vi "Client.vi"() -> ()   [LabVIEW 2020]
panel:
  out "Data transmise":string
  out "bytes written 2":i32
  in  "Port distant":u16
  out "bytes written":i32
  in  "Vit":dbl(slide) scale=-1.0..1.0
  in  "stop":bool
  out "error out":errorcluster
  # "Client"
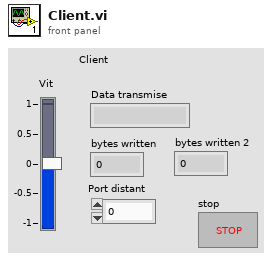
[diagram p1: front panel]
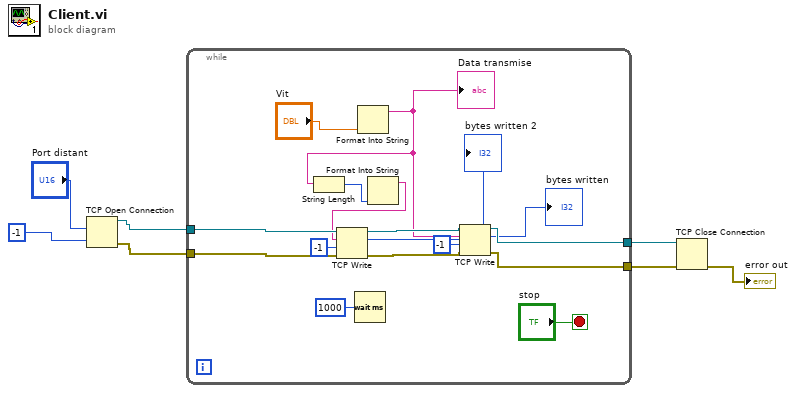
[diagram p0: block diagram]
diagram:
  n1 = TCP Open Connection(remote port or service name="Port distant", timeout ms (60000)=-1 ("timeout ms (wait forever: -1)")) -> (connection ID=w3:refnum<k5>, error out=w2:errorcluster)  [unwired: 3 in]
  n2 = while {
    tunnel: w3 -> [w21]
    tunnel: [w17] -> w7
    tunnel: w2 -> [w20]
    tunnel: [w18] -> w6
    stop <- "stop" stop-if-true
    n3 = Wait (ms)(milliseconds to wait=u32 1000) -> ()  [unwired: 1 out]
    n4 = Format Into String("Vit") -> (resulting string=w15:string)  [unwired: 3 in, 1 out]
    "Data transmise" <- w15
    n5 = String Length(string=w15) -> (length=w14:i32)
    n6 = Format Into String(w14) -> (resulting string=w8:string)  [unwired: 3 in, 1 out]
    n7 = TCP Write(connection ID=w21, data in=w8, error in (no error)=w20, 9:-1 ("timeout ms (25000)")) -> (connection ID out=w16:refnum<k5>, bytes written=→"bytes written 2":i32, error out=w19:errorcluster)
    n8 = TCP Write(connection ID=w16, data in=w15, error in (no error)=w19, 9:-1 ("timeout ms (25000)")) -> (connection ID out=w17:refnum<k5>, bytes written=→"bytes written":i32, error out=w18:errorcluster)
  }
  n9 = TCP Close Connection(connection ID=w7, error in (no error)=w6) -> (error out=→"error out":errorcluster)  [unwired: 1 in, 1 out]
